vi "Receiver_Example_Img - Copy.vi"() -> ()   [LabVIEW 2018]
uses:
  <vilib>/picture/picture.llb/imagedata.ctl
panel:
  out "Panjang data 2":i32
  out "Modulation parameter 2":T1
  out "Array":i32[](array[numeric])
  out "x/y 3":dbl
  out "size(s) 3":i32
  out "size(s) 2":i32
  out "x/y 2":dbl
  out "Numeric":i32
  out "output ditransmisikan":i16[](array[numeric])
  out "0, 1":i16[][](array[numeric])
  out "1-bit pixmap":bool[][](array[boolean])
  out "new picture":picture
  out "image data":T2
  in  "path to BMP file":path=path "D:/Thesis Pak Pri/pict.bmp"
  out "output array":i32[][](array[numeric])
  out "output diterima":bool[][](array[boolean])
  out "Gambar Terima":picture
  in  "Width":i32=256
  in  "Height":i32=256
  out "x/y":dbl
  out "x > y?":bool
  out "size(s)":i32
  out "output bits":i8[](array[numeric])
  in  "Panjang data":i32=3600
  out "sisa bagi":i32
  out "hasil bagi":i32
  out "iterasi":i32
  in  "String":string="PENS"
  in  "Modulation parameter":T1
  out "created new?":bool
  out "XY Graph":cdb[](graph)
  out "SIG valid?":bool
  out "Frequency offset":dbl
  in  "stop":bool
  out "USRP CoercedParamters":T3={"coerced IQ rate"=100000.0, "coerced carrier frequency"=100000.0, "coerced gain"=0.0} {"coerced gain" format="%#_6f"; "coerced carrier frequency" format="%#_6p"; "coerced IQ rate" format="%#_6p"}
  out "error out":errorcluster
  in  "Trigger level":dbl=0.005 format="%f"
  in  "error in (no error)":errorcluster
  in  "USRP ControledParameters":T4={"active antenna"="RX1", "gain"=0.0, "carrier frequency"=915000000.0, "IQ rate"=1000000.0} {"IQ rate" format="%#_6p"; "carrier frequency" format="%#_6p"; "gain" format="%#_6f"}
  in  "device names":refnum<k15>="192.168.10.4"
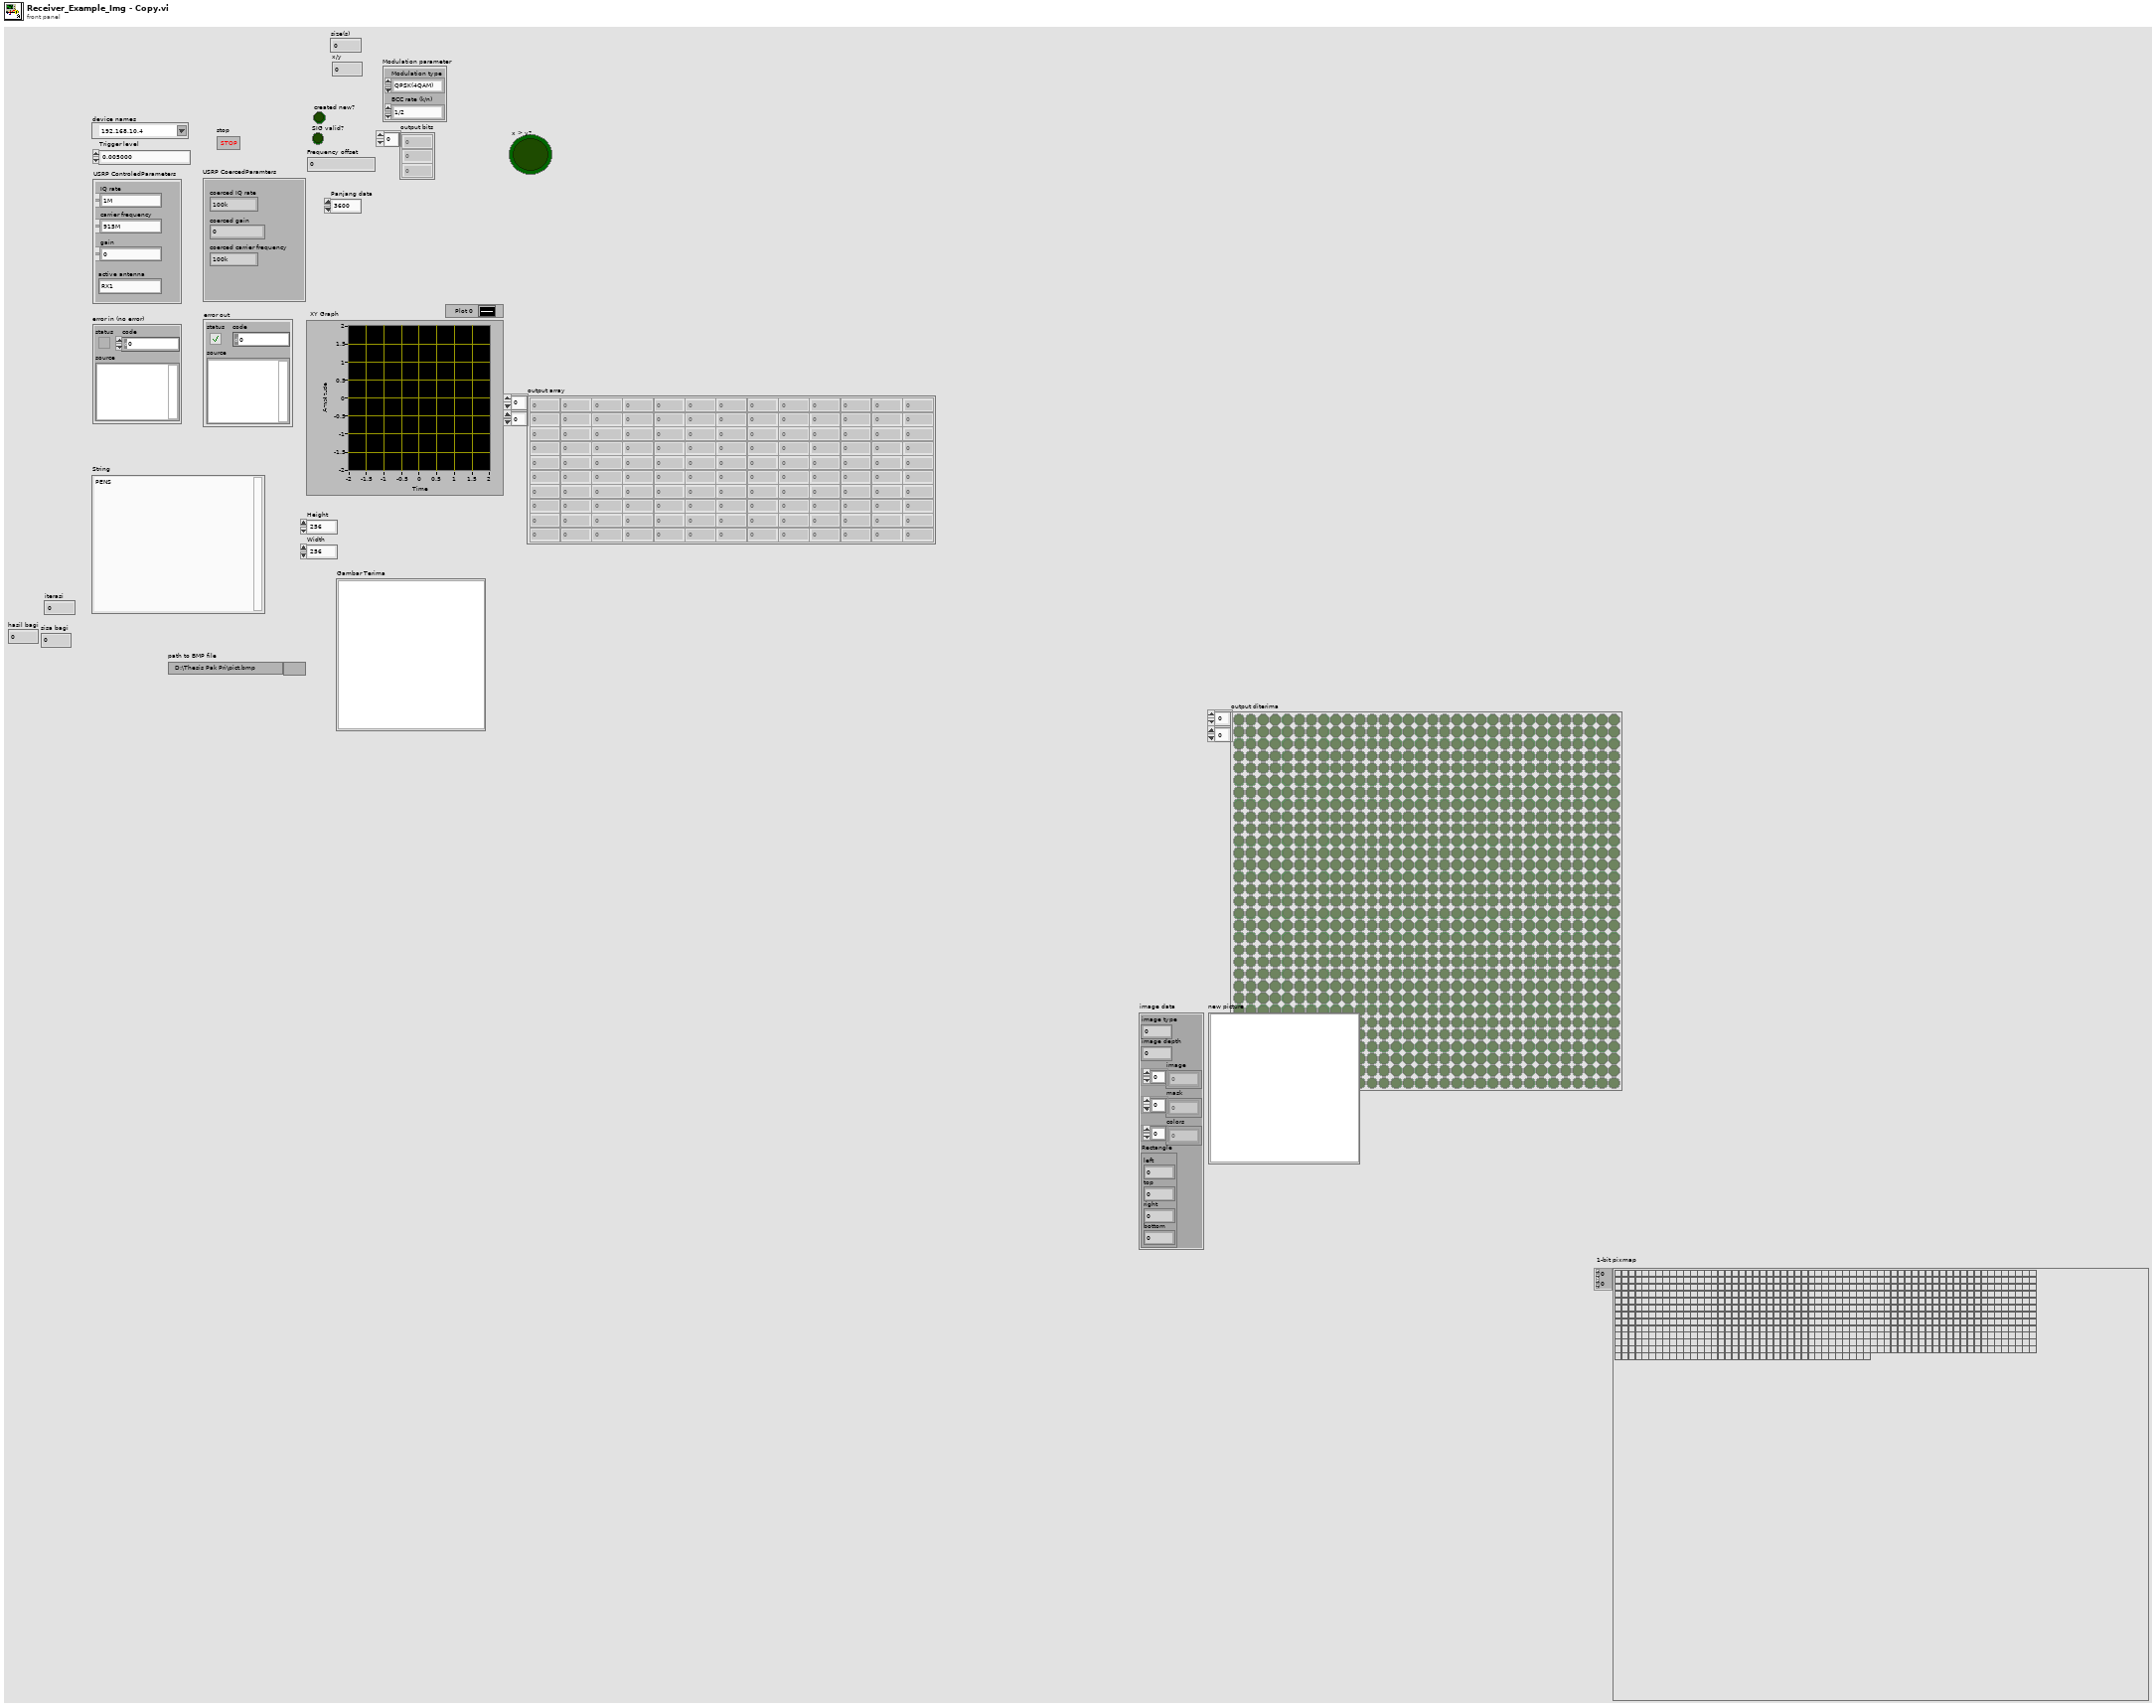
[diagram p1: front panel]
types:
  T1 = cluster{"Modulation type":enum16{"QPSK(4QAM)", "64QAM", "16QAM", "BPSK"}, "BCC rate (k/n)":enum16{"1/2", "2/3", "3/4"}}
  T2 = typedef "imagedata.ctl" = cluster{"image type":i32, "image depth":i32, "image":u8[], "mask":u8[], "colors":u32[], "Rectangle":cluster{"left":i16, "top":i16, "right":i16, "bottom":i16}}
  T3 = cluster{"coerced IQ rate":dbl, "coerced carrier frequency":dbl, "coerced gain":dbl}
  T4 = cluster{"active antenna":string, "gain":dbl, "carrier frequency":dbl, "IQ rate":dbl}
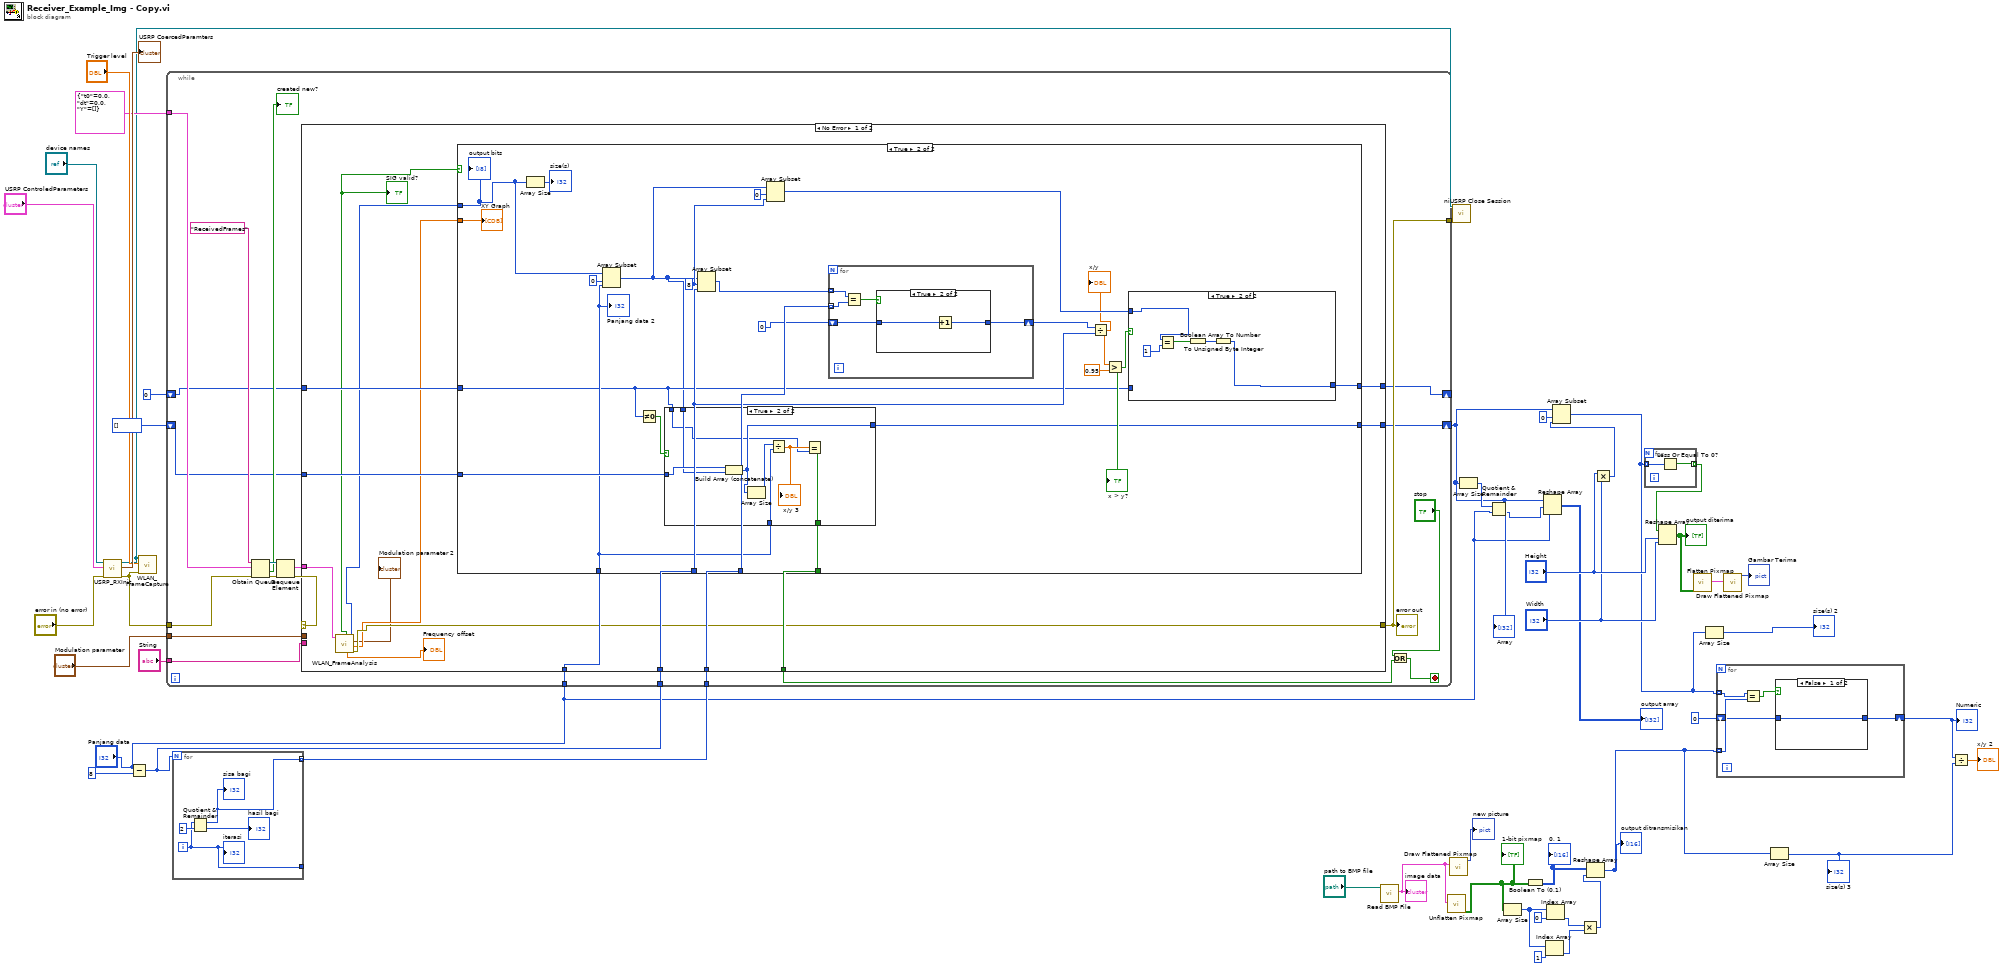
[diagram p0: block diagram]
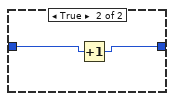
[diagram p2: hidden frame]
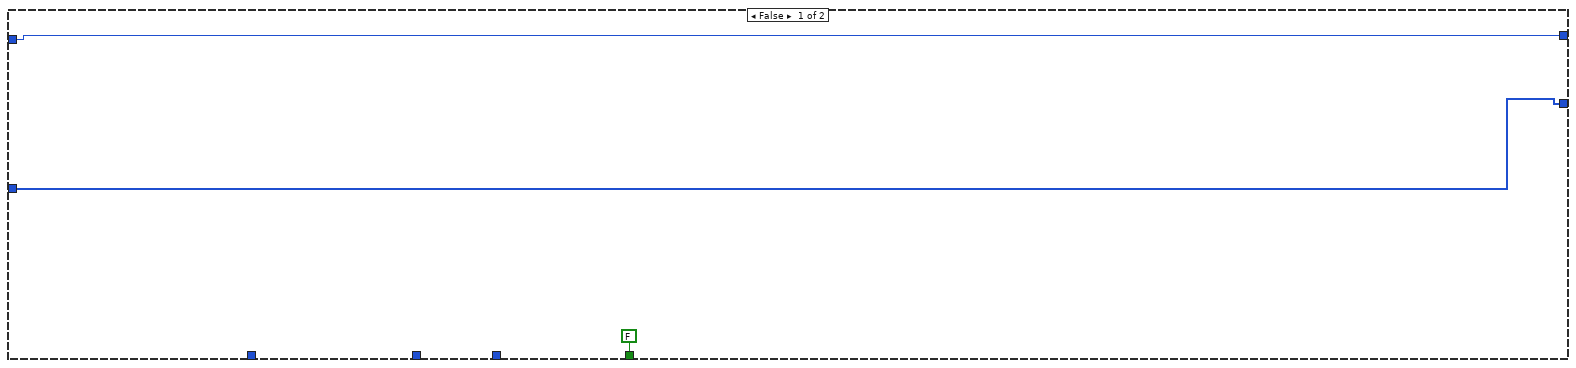
[diagram p3: hidden frame]
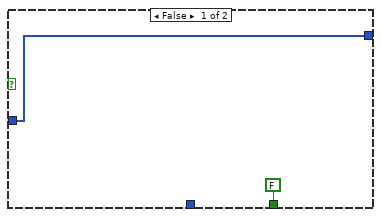
[diagram p4: hidden frame]
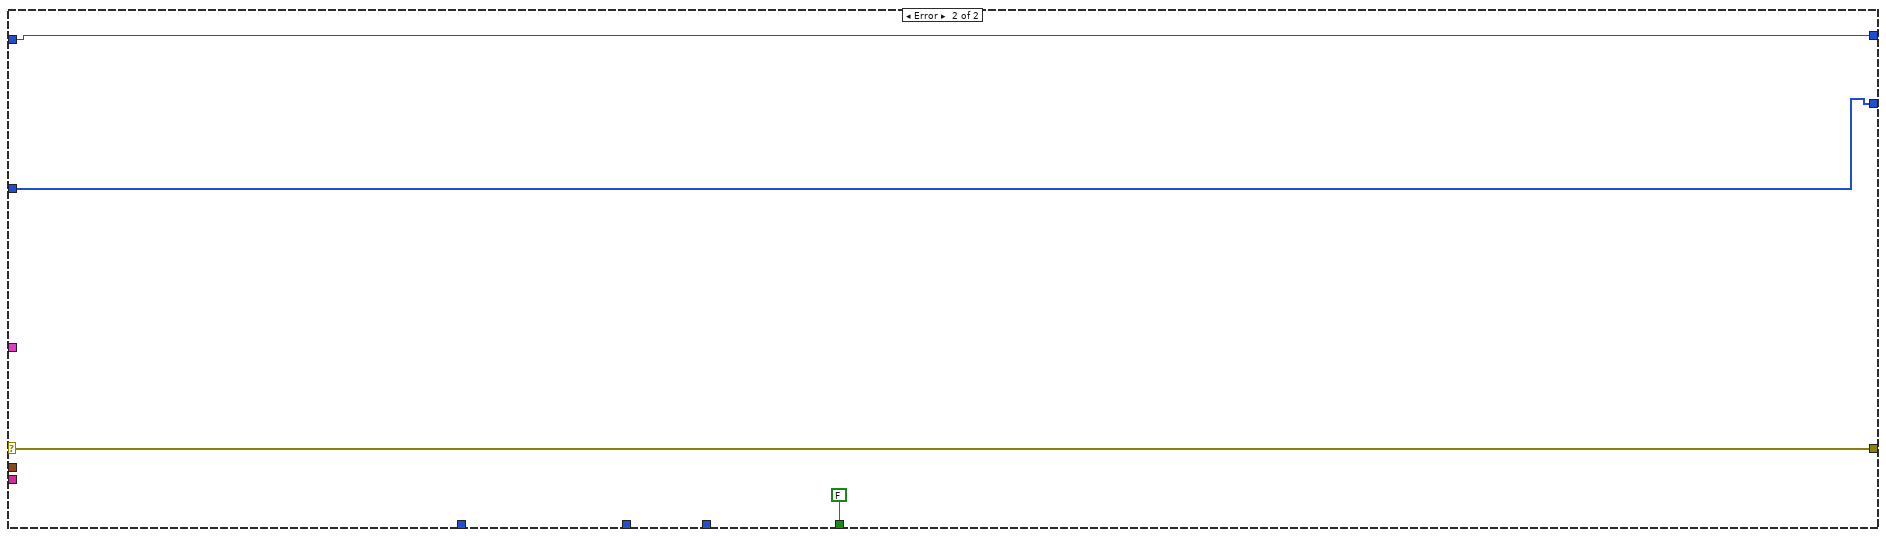
[diagram p7: hidden frame]
diagram:
  n1 = call "USRP_RXInit.vi"("device names"="device names", "USRP ControledParameters"="USRP ControledParameters", "error in (no error)"="error in (no error)") -> ("session handle out"=w39:refnum<k15>, "USRP CoercedParamters"=→"USRP CoercedParamters":T3, "error out"=w43:errorcluster)  [unwired: 5 in]
  n2 = Subtract(x="Panjang data", y=8) -> (x-y=w35:i32)
  n3 = call "WLAN_FrameCapture.vi"("error in (no error)"=w43, "Trigger level"="Trigger level", "session handle"=w39) -> ()  [unwired: 8 in]
  n4 = for {
    N: w35 -> [_]
    tunnel: [w49] -> _
    tunnel: [w48] -> w34 mode=indexing
    i -> [w49]
    n5 = Quotient & Remainder(x=w49, y=2) -> (x-y*floor(x/y)=w48:i32, floor(x/y)=→"hasil bagi":i32)
    "sisa bagi" <- w48
    "iterasi" <- w49
  }
  n6 = while {
    tunnel: w43 -> [w71]
    tunnel: cluster{"t0":dbl, "dt":dbl, "Y":cdb[]} {"t0"=0.0, "dt"=0.0, "Y"=[]} ("data") -> [w72]
    tunnel: [w64] -> w40
    tunnel: "Modulation parameter" -> [w63]
    tunnel: "String" -> [w62]
    tunnel: "Panjang data" -> [w61]
    tunnel: w35 -> [w60]
    tunnel: w34 -> [w59]
    shift-right: [w57] -> _
    shift-left: 0 -> [w58]
    shift-right: [w55] -> w23
    shift-left: i32[] [] -> [w56]
    stop <- w52 stop-if-true
    n7 = Obtain Queue(name (unnamed)="ReceivedFrames", element data type=w72, error in (no error)=w71) -> (queue out=w70:refnum<queue>, created new?=→"created new?":bool, error out=w67:errorcluster)  [unwired: 2 in]
    n8 = Dequeue Element(queue=w70, error in (no error)=w67) -> (element=w68:cluster{"t0":dbl, "dt":dbl, "Y":cdb[]}, error out=w69:errorcluster)  [unwired: 1 in, 2 out]
    n9 = case shown="No Error" w69 {
      selector: w69 -> [_ w141]
      tunnel: w68 -> [w79 _]
      tunnel: [w78 w141] -> w64
      tunnel: w63 -> [_ _]
      tunnel: w62 -> [_ _]
      tunnel: w61 -> [w87 _]
      tunnel: w60 -> [w86 _]
      tunnel: w59 -> [w85 _]
      tunnel: w58 -> [w84 w140]
      tunnel: [w83 w140] -> w57
      tunnel: w56 -> [w82 w139]
      tunnel: [w81 w139] -> w55
      tunnel: [w80 FALSE] -> w53
      frame No Error {
        n10 = call "WLAN_FrameAnalysis.vi"("input cluster"=w79) -> ("error out"=w78:errorcluster, "Constellation"=w74:cdb[], "Modulation parameter"=→"Modulation parameter 2":T1, "output bits"=w76:i8[], "Frequency offset"=→"Frequency offset":dbl, "SIG valid?"=w77:bool)  [unwired: 5 in]
        "SIG valid?" <- w77
        n11 = case shown="True" w77 {
          tunnel: w76 -> [_ w91]
          tunnel: w74 -> [_ w113]
          tunnel: w87 -> [_ w97]
          tunnel: w86 -> [_ w106]
          tunnel: w85 -> [_ w109]
          tunnel: w84 -> [w90 w96]
          tunnel: [w90 w100] -> w83
          tunnel: w82 -> [w89 w98]
          tunnel: [w89 w94] -> w81
          tunnel: [FALSE w95] -> w80
          frame False {
          }
          frame True {
            w102 = 8 ("index")
            n12 = Array Size(array=w91) -> (size(s)=→"size(s)":i32)
            n13 = Array Subset(array=w91, index=0, length=w97) -> (w92:i8[])
            n14 = Not Equal To 0?(x=w96) -> (x != 0?=w99:bool)
            n15 = case shown="True" w99 {
              tunnel: w98 -> [w115 w123]
              tunnel: w92 -> [_ w122]
              tunnel: [w115 w119] -> w94
              tunnel: w97 -> [_ w118]
              tunnel: w96 -> [_ w117]
              tunnel: [FALSE w116] -> w95
              frame False {
              }
              frame True {
                n16 = Build Array (concatenate)(w123, w122) -> (w119:i32[])
                n17 = Array Size(array=w119) -> (size(s)=w121:i32)
                n18 = Divide(x=w121, y=w118) -> (x/y=w120:dbl)
                "x/y 3" <- w120
                n19 = Equal?(x=w120, y=w117) -> (x = y?=w116:bool)
              }
            }
            n20 = Array Subset(array=w92, index=w102, length=w106) -> (w110:i8[])
            n21 = Array Subset(array=w92, index=0, length=w102) -> (w101:i8[])
            n22 = for {
              tunnel: w110 -> [w133] mode=indexing
              tunnel: w109 -> [w134] mode=indexing
              shift-right: [w130] -> w107
              shift-left: 0 -> [w131]
              n23 = Equal?(x=w133, y=w134) -> (x = y?=w132:bool)
              n24 = case shown="True" w132 {
                tunnel: w131 -> [w135 w137]
                tunnel: [w135 w136] -> w130
                frame False {
                }
                frame True {
                  n25 = Increment(x=w137) -> (x+1=w136:i32)
                }
              }
            }
            n26 = Divide(x=w107, y=w106) -> (x/y=w93:dbl)
            "x/y" <- w93
            n27 = Greater?(x=w93, y=0.95) -> (0:w104:bool)
            "x > y?" <- w104
            n28 = case shown="True" w104 {
              tunnel: w101 -> [_ w127]
              tunnel: w96 -> [w124 _]
              tunnel: [w124 w125] -> w100
              frame False {
              }
              frame True {
                n29 = Equal?(x=w127, y=1) -> (x = y?=w128:bool[])
                n30 = Boolean Array To Number(Boolean array=w128) -> (number=w126:u32)
                n31 = To Unsigned Byte Integer(number=w126) -> (unsigned 8bit integer=w125:u8)
              }
            }
            "XY Graph" <- w113
            "output bits" <- w91
            "Panjang data 2" <- w97
          }
        }
      }
      frame Error {
      }
    }
    "error out" <- w64
    n32 = Or(x="stop", y=w53) -> (x .or. y?=w52:bool)
  }
  "Array" <- w23
  n33 = call <vilib>:"Read BMP File.vi"("path to BMP file"="path to BMP file") -> ("image data"=w17:T2)  [unwired: 8 in, 2 out]
  "image data" <- w17
  n34 = call <vilib>:"Unflatten Pixmap.vi"("image data"=w17) -> ("1-bit pixmap"=w15:bool[][])  [unwired: 4 in, 6 out]
  "1-bit pixmap" <- w15
  n35 = call <vilib>:"Draw Flattened Pixmap.vi"("image data"=w17) -> ("new picture"=→"new picture":picture)  [unwired: 8 in]
  n36 = call <instrlib>:"niUSRP Close Session.vi"("session handle"=w39, "error in (no error)"=w40) -> ()  [unwired: 13 in, 1 out]
  n37 = Array Size(array=w23) -> (size(s)=w31:i32)
  n38 = Quotient & Remainder(x=w31, y="Panjang data") -> (floor(x/y)=w22:i32)  [unwired: 1 out]
  n39 = Array Size(array=w15) -> (size(s)=w12:i32[])
  n40 = Boolean To (0,1)(Boolean=w15) -> (0, 1=w16:i16[][])
  "0, 1" <- w16
  n41 = Reshape Array(w23, w22, "Panjang data") -> (→"output array":i32[][])
  n42 = Index Array(array=w12, index=1) -> (element=w10:i32)
  n43 = Index Array(array=w12, index=0) -> (element=w11:i32)
  n44 = Multiply(x=w11, y=w10) -> (x*y=w9:i32)
  n45 = Reshape Array(w16, w9) -> (w7:i16[])
  "output ditransmisikan" <- w7
  n46 = Multiply(x="Height", y="Width") -> (x*y=w24:i32)
  n47 = Array Subset(array=w23, index=0, length=w24) -> (w3:i32[])
  n48 = for {
    tunnel: w3 -> [w143] mode=indexing
    tunnel: [w142] -> w29 mode=indexing
    n49 = Less Or Equal To 0?(x=w143) -> (x <= 0?=w142:bool)
  }
  n50 = Reshape Array(w29, "Height", "Width") -> (w28:bool[][])
  "output diterima" <- w28
  n51 = call <vilib>:"Flatten Pixmap.vi"("1-bit pixmap"=w28) -> ("image data"=w30:T2)  [unwired: 10 in]
  n52 = Array Size(array=w3) -> (size(s)=→"size(s) 2":i32)
  n53 = for {
    tunnel: w3 -> [w148] mode=indexing
    tunnel: w7 -> [w147] mode=indexing
    shift-right: [w144] -> w6
    shift-left: 0 -> [w145]
    n54 = Equal?(x=w148, y=w147) -> (x = y?=w146:bool)
    n55 = case shown="False" w146 {
      tunnel: w145 -> [w149 w151]
      tunnel: [w149 w150] -> w144
      frame False {
      }
      frame True {
        n56 = Increment(x=w151) -> (x+1=w150:i32)
      }
    }
  }
  "Numeric" <- w6
  n57 = call <vilib>:"Draw Flattened Pixmap.vi"("image data"=w30) -> ("new picture"=→"Gambar Terima":picture)  [unwired: 8 in]
  n58 = Array Size(array=w7) -> (size(s)=w5:i32)
  "size(s) 3" <- w5
  n59 = Divide(x=w6, y=w5) -> (x/y=→"x/y 2":dbl)
